vi "AudioTest.Audio Test, Detect Devices.vi"(8 "error in (no error)":errorcluster, 9 "UUT is Mic(F)\\Speaker(T)":bool, 10 "Mic Device":string, 11 "Speaker Device":string) -> (0 "error out":errorcluster)   [LabVIEW 2018]
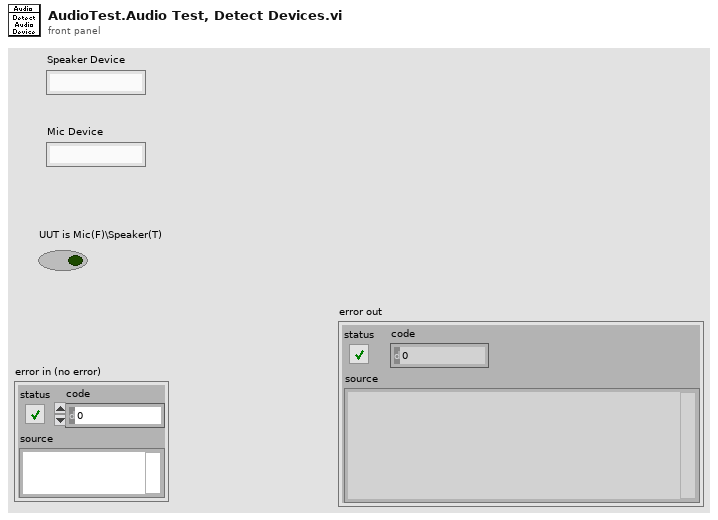
[diagram p1: front panel]
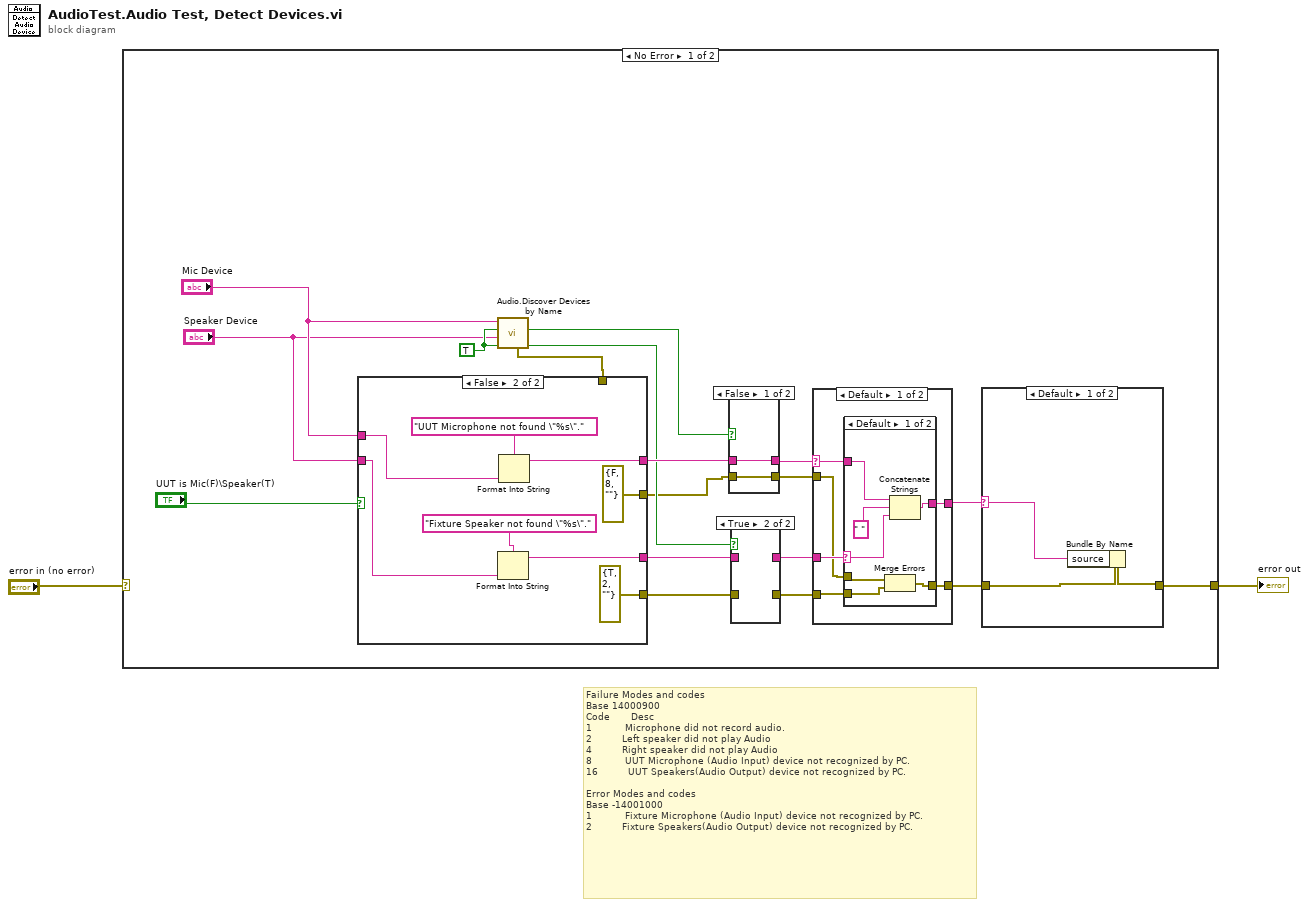
[diagram p0: block diagram]
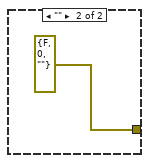
[diagram p2: hidden frame]
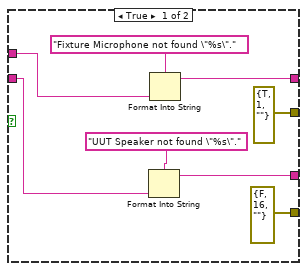
[diagram p7: hidden frame]
diagram:
  # "Failure Modes and codes\nBase 14000900\nCode       Desc\n1           Microphone did not record audio.\n2          Left speaker did not play Audio\n4          Right speaker did not play Audio\n8           UUT Microphone (Audio Input) device not recognized by PC.\n16          UUT Speakers(Audio Output) device not recognized by PC.\n\nError Modes and codes\nBase -14001000\n1           Fixture Microphone (Audio Input) device not recognized by PC.\n2          Fixture Speakers(Audio Output) device not recognized by PC."
  n1 = case shown="No Error" "error in (no error)" {
    selector: "error in (no error)" -> [_ w62]
    tunnel: [w9 w62] -> w1
    frame No Error {
      w20 = TRUE ("Error if In Dev Not Found")
      n2 = call "Audio.Discover Devices by Name.vi"("Error if Out Dev Not Found"=w20, "Output Device"="Speaker Device", "Error if In Dev Not Found"=w20, "Input Device"="Mic Device") -> ("Out Dev Found"=w14:bool, "In Dev Found"=w16:bool, "error out"=w3:errorcluster)  [unwired: 3 in, 2 out]
      n3 = case shown="False" "UUT is Mic(F)\\Speaker(T)" {
        tunnel: "Mic Device" -> [w52 w60]
        tunnel: "Speaker Device" -> [w51 w59]
        tunnel: [w49 w57] -> w13
        tunnel: [w48 w56] -> w15
        tunnel: [errorcluster {"status"=TRUE, "code"=1, "source"=""} ("error constant") errorcluster {"status"=FALSE, "code"=8, "source"=""} ("error constant")] -> w8
        tunnel: [errorcluster {"status"=FALSE, "code"=16, "source"=""} ("error constant") errorcluster {"status"=TRUE, "code"=2, "source"=""} ("error constant")] -> w6
        tunnel: w3 -> [_ _]
        frame True {
          n4 = Format Into String(format string="UUT Speaker not found \"%s\".", w51) -> (resulting string=w49:string)  [unwired: 2 in, 1 out]
          n5 = Format Into String(format string="Fixture Microphone not found \"%s\".", w52) -> (resulting string=w48:string)  [unwired: 2 in, 1 out]
        }
        frame False {
          n6 = Format Into String(format string="Fixture Speaker not found \"%s\".", w59) -> (resulting string=w57:string)  [unwired: 2 in, 1 out]
          n7 = Format Into String(format string="UUT Microphone not found \"%s\".", w60) -> (resulting string=w56:string)  [unwired: 2 in, 1 out]
        }
      }
      n8 = case shown="False" w16 {
        tunnel: w15 -> [w45 _]
        tunnel: [w45 _] -> w12
        tunnel: w8 -> [w44 _]
        tunnel: [w44 _] -> w7
        frame False {
        }
        frame True {
        }
      }
      n9 = case shown="True" w14 {
        tunnel: w13 -> [w43 _]
        tunnel: [w43 _] -> w11
        tunnel: w6 -> [w42 _]
        tunnel: [w42 _] -> w5
        frame False {
        }
        frame True {
        }
      }
      n10 = case shown="Default" w12 {
        selector: w12 -> [w28 _]
        tunnel: w11 -> [w30 w41]
        tunnel: [w29 w41] -> w10
        tunnel: w7 -> [w27 _]
        tunnel: w5 -> [w26 w40]
        tunnel: [w25 w40] -> w4
        frame Default {
          n11 = case shown="Default" w30 {
            selector: w30 -> [w34 _]
            tunnel: [w37 w39] -> w29
            tunnel: w28 -> [w36 w39]
            tunnel: w27 -> [w33 w38]
            tunnel: w26 -> [w32 _]
            tunnel: [w31 w38] -> w25
            frame Default {
              n12 = Merge Errors(w33, w32) -> (w31:errorcluster)
              n13 = Concatenate Strings(w36, " ", w34) -> (w37:string)
            }
            frame "" {
            }
          }
        }
        frame "" {
        }
      }
      n14 = case shown="Default" w10 {
        selector: w10 -> [w21 _]
        tunnel: [w23 errorcluster {"status"=FALSE, "code"=0, "source"=""} ("error constant")] -> w9
        tunnel: w4 -> [w22 _]
        frame Default {
          n15 = Bundle By Name(cluster=w22, "source"=w21) -> (w23:errorcluster)
        }
        frame "" {
        }
      }
    }
    frame Error {
    }
  }
  "error out" <- w1
